vi "Tosca-Save State.vi"(0 "State":T1, 11 "Error In":errorcluster) -> (15 "Error Out":errorcluster)   [LabVIEW 2020]
uses:
  Typedefs/Tosca-State.ctl
  Typedefs/Tosca-Thread Type.ctl
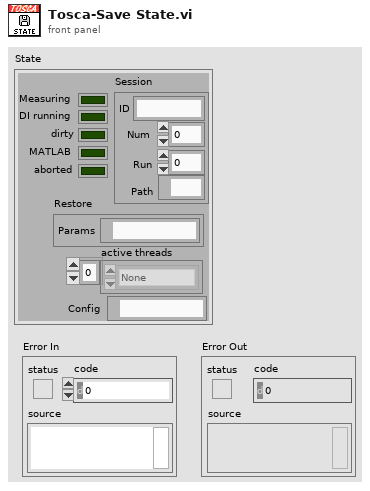
[diagram p1: front panel]
types:
  T1 = typedef "Tosca-State.ctl" = cluster{"Measuring":bool, "DI running":bool, "dirty":bool, "Restore":cluster{"Params":path}, "Session":cluster{"ID":string, "Num":i32, "Path":path, "Run":i32}, "active threads":T2[], "MATLAB":bool, "Config":path, "aborted":bool}
  T2 = typedef "Tosca-Thread Type.ctl" = enum16{"None", "AODO", "Masker", "ET", "Imaging", "Pupil", "AI", "DI", "Camera", "TTL out", "Loco", "Visual"}
  T3 = cluster{"ID":string, "Num":i32, "Path":path, "Run":i32}
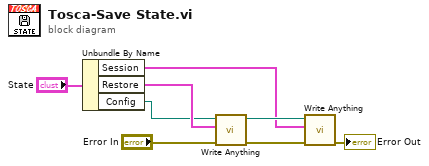
[diagram p0: block diagram]
diagram:
  n1 = Unbundle By Name("State") -> ("Session"=w3:T3, "Restore"=w2:cluster{"Params":path}, "Config"=w1:path)
  n2 = call "Write Anything.vi"("Error In"="Error In", "Anything"=w2, "Path (dialog)"=w1) -> ("Error Out"=w6:errorcluster, "Path out"=w8:path)  [unwired: 7 in]
  n3 = call "Write Anything.vi"("Error In"=w6, "Anything"=w3, "Path (dialog)"=w8) -> ("Error Out"=→"Error Out":errorcluster)  [unwired: 7 in, 1 out]
